vi "Dashboard Main.vi"() -> ()   [LabVIEW 2018]
uses:
  <vilib>/Rock Robotics/WPI/Camera/WPI_CameraExposure Values.ctl
  <vilib>/Rock Robotics/WPI/Camera/WPI_CameraWhite Balance Values.ctl
  <vilib>/Utility/miscctls.llb/LVRowAndColumnTypeDef.ctl
  <vilib>/event_ctls.llb/eventvkey.ctl
  <vilib>/Rock Robotics/Network Tables/NT Read Numeric Array.vi
  <vilib>/Rock Robotics/WPI/Dashboard/WPI_DashboardLogging Global.vi
  Dashboard globals.vi
  <vilib>/vision/NI_Vision_Development_Module.lvlib
panel:
  in  "Camera Settings Right":T1={"Frame Rate"=30, "Compression"=30, "Size"=1, "DB Camera Config"=FALSE} {"Frame Rate" scale=1.0..30.0; "Compression" scale=100.0..-1.0; "Size" items=["640x480", "320x240", "160x120"]}
  in  "Camera Name Right":string(combo)="No Camera Selection"
  out "Camera Perf":string
  in  "Camera Settings":T1={"Frame Rate"=30, "Compression"=30, "Size"=1, "DB Camera Config"=FALSE} {"Frame Rate" scale=1.0..30.0; "Compression" scale=100.0..-1.0; "Size" items=["640x480", "320x240", "160x120"]}
  in  "TCP":refnum<k5>
  in  "Rec Mode":enum32{"Stop", "Record", "Playback"}(radio)
  out "Robot IP":string
  out "Image Message":string="Timeout in Camera Communications"
  in  "Dashboard Tab":T2(tab)=enum."Custom"
  in  "Reset":bool
  out "Total Stored\nSince Reset":i32
  in  "# New Images\nto Store":i32=1
  in  "Photo\nStore Rate":u32=100
  in  "Start\nStoring":bool
  in  "Select Auto":string(combo)="Select Autonomous ..."
  out "NT Connection":bool
  out "MotorChart R":cluster{"Numeric":dbl, "Numeric":dbl}(graph)
  out "MotorChart L":cluster{"Numeric":dbl, "Numeric":dbl}(graph)
  out "MotorSliders R":cluster{"MotorSlide1":dbl, "MotorSlide2":dbl} {"MotorSlide2" scale=-1.0..1.0 scale format="%#_2e"; "MotorSlide1" scale=-1.0..1.0 scale format="%#_2e"}
  out "MotorSliders L":cluster{"MotorSlide1":dbl, "MotorSlide2":dbl} {"MotorSlide2" scale=-1.0..1.0 scale format="%#_2e"; "MotorSlide1" scale=-1.0..1.0 scale format="%#_2e"}
  out "Gyro":dbl(knob) scale=0.0..360.0
  out "JS1 Z":dbl(slide) scale=-1.0..1.0 scale format="%#_2e"
  out "JS1 Graph":cluster{"X":dbl, "Y":dbl}[](graph)
  out "JS1 Buttons":T3
  out "JS2 Z":dbl(slide) scale=-1.0..1.0 scale format="%#_2e"
  out "JS2 Graph":cluster{"X":dbl, "Y":dbl}[](graph)
  out "JS2 Buttons":T3
  out "Mode":T4(ring)=enum."Auto Disabled"
  out "Right Camera Perf":cluster{"Bandwidth (Mbps)":dbl, "FPS":dbl}
  out "Camera Image Right":T5(plugin-control)
  in  "DB/String 9":string
  in  "DB/String 8":string
  in  "DB/String 7":string
  in  "DB/String 6":string
  in  "DB/String 5":string
  in  "DB/String 4":string
  in  "DB/String 3":string
  in  "DB/String 2":string
  in  "DB/String 1":string
  in  "DB/String 0":string
  in  "DB/Slider 0":dbl(slide) scale=0.0..5.0
  in  "DB/Slider 1":dbl(slide) scale=0.0..5.0
  in  "DB/Slider 2":dbl(slide) scale=0.0..5.0
  in  "DB/Slider 3":dbl(slide) scale=0.0..5.0
  out "DB/LED 3":bool
  out "DB/LED 2":bool
  out "DB/LED 1":bool
  out "DB/LED 0":bool
  in  "DB/Button 3":bool
  in  "DB/Button 2":bool
  in  "DB/Button 1":bool
  in  "DB/Button 0":bool caption="New Name"
  out "Right width":sgl
  out "Left width":sgl
  out "Right y":sgl
  out "Right x":sgl
  out "Left y":sgl
  out "Left x":sgl
  out "Right height":sgl
  out "Left height":sgl
  in  "Desired Target":T6(radio)=enum."Ship Right"
  in  "Enable Vision\nProcessing":bool
  in  "Test Slider":dbl(slide) scale=0.0..100.0 scale format="%#_3g"
  in  "On/Off":bool caption="Solenoid"
  in  "Test Name":u16(ring) items=["Select the test to run..."]
  in  "Test Tree":string(tree)
  in  "Motor":cluster{"Value":dbl, "Enable":bool} {"Value" scale=-1.0..1.0 scale format="%#_3g"}
  out "Progress":T7 {"Test Progress" scale=0.0..100.0}
  in  "Rev/Fwd":cluster{"Forward":bool, "Reverse":bool}
  in  "Test Ring":u16(ring) items=["Monochrome", "Color"]
  out "Cmd Status":string
  in  "Execute Command":bool
  in  "Command Params":string[][](table)
  in  "Command Selection":i32(listbox)
  in  "CheckList":i32(listbox)
  out "Tree":string(tree)
  out "Camera Image":T5(plugin-control)
  out "Background":bool
  in  "Camera Name":string(combo)="No Camera Selection"
  # "HW"
  # "HW"
  # "Joysticks"
  # "Drive Motors"
  # "Front"
  # "Right"
  # "Left"
  # "Back"
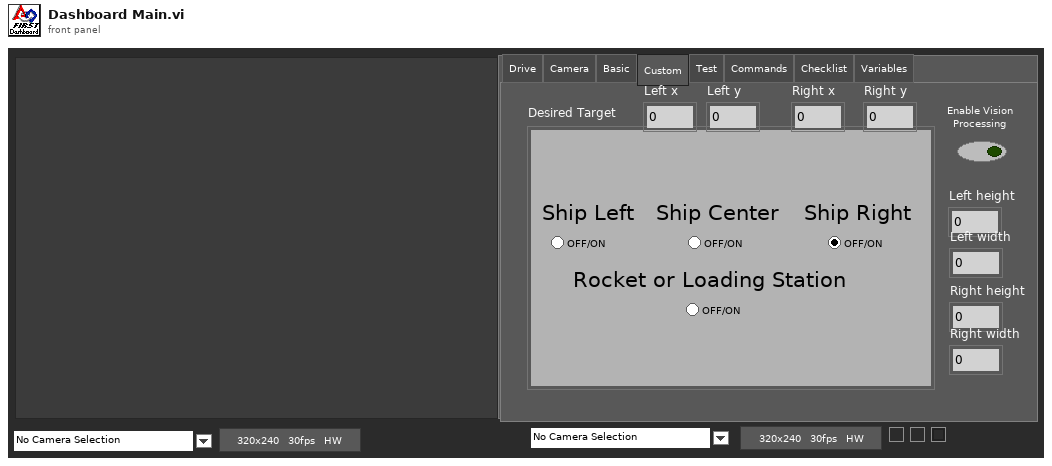
[diagram p1: front panel]
types:
  T1 = cluster{"Frame Rate":i32, "Compression":i32, "Size":u16, "DB Camera Config":bool}
  T2 = enum32{"Drive", "Camera", "Basic", "Custom", "Test", "Commands", "Checklist", "Variables"}
  T3 = cluster{bool, bool, bool, bool, bool, bool, bool, bool, bool, bool, bool, bool}
  T4 = enum8{"Tele-Op Disabled", "Tele-Op Enabled", "Auto Disabled", "Auto Enabled", "Test Disabled", "Test Enabled", "Disconnected", "No Code", "E-Stop"}
  T5 = typedef "IMAQ Image.ctl" = refnum<image>
  T6 = enum32{"Ship Left", "Ship Center", "Ship Right", "Rocket or Loading Station"}
  T7 = cluster{"Test Progress":u8, "Test Progress Text":string}
  T8 = cluster{"Save Path":path, "Interval (s)":dbl, "Keep":i32}
  T9 = typedef "Image Type" = u32
  T10 = cluster{"IDs":cluster{"RPC field ID":u16, "Unique ID":u16}, "String":string}
  T11 = cluster{"Camera Image":refnum<vi>, "Dashboard Tab":refnum<vi>, "Background":refnum<vi>, "Rec Mode":refnum<vi>, "Test Slider":refnum<vi>, "On/Off ":refnum<vi>, "Test Ring":refnum<vi>, "Rev/Fwd":refnum<vi>, "Test Name":refnum<vi>, "Motor":refnum<vi>, "Progress":refnum<vi>, "CheckList":refnum<vi>, "Tree":refnum<vi>, "Test Tree":refnum<vi>, "Command Params":refnum<vi>, "Command Selection":refnum<vi>, "Execute Command":refnum<vi>, "Cmd Status":refnum<vi>, "Camera Settings":refnum<vi>, "Camera Name":refnum<vi>, "Camera Perf":refnum<vi>, "Camera Settings Right":refnum<vi>, "Camera Name Right":refnum<vi>, "Camera Image Right":refnum<vi>}
  T12 = typedef "WPI_CameraExposure Values.ctl" = enum16{"Auto", "Flicker-free 50 Hz", "Flicker-free 60 Hz", "Hold current", "Custom"}
  T13 = typedef "WPI_CameraWhite Balance Values.ctl" = enum16{"Auto", "Fixed indoor", "Fixed outdoor 1", "Fixed outdoor 2", "Fixed fluorescent 1", "Fixed fluorescent 2", "Hold current", "Custom"}
  T14 = cluster{"Exposure":T12, "Exposure (%)":dbl, "Brightness":i32, "White Balance":T13, "Color Temp (K)":dbl}
  T15 = cluster{"Global Rectangle":i32[], "Contours":cluster{"Contour Type":u32, "ROI Type":u32, "Points":i32[]}[]}
  T16 = cluster{"Corners":cluster{"X":sgl, "Y":sgl}[], "Orientation (degrees)":dbl, "Width":dbl, "Height":dbl, "Score":dbl}[]
  T17 = cluster{"Camera Name":string, string, "Saved DB Images Info":cluster{"Save Path":path, "Interval (s)":dbl, "Keep":i32}}
  T18 = cluster{"Corners":cluster{"X":sgl, "Y":sgl}[], "Orientation (degrees)":dbl, "Width":dbl, "Height":dbl, "Score":dbl}
  T19 = cluster{"Corners[0]":cluster{"X":sgl, "Y":sgl}, "Corners[1]":cluster{"X":sgl, "Y":sgl}, "Corners[2]":cluster{"X":sgl, "Y":sgl}, "Corners[3]":cluster{"X":sgl, "Y":sgl}, "Corners[4]":cluster{"X":sgl, "Y":sgl}, "Corners[5]":cluster{"X":sgl, "Y":sgl}, "Corners[6]":cluster{"X":sgl, "Y":sgl}, "Corners[7]":cluster{"X":sgl, "Y":sgl}, "Corners[8]":cluster{"X":sgl, "Y":sgl}}
  T20 = cluster{"Camera Name Right":string, string, "Saved DB Images Info":cluster{"Save Path":path, "Interval (s)":dbl, "Keep":i32}}
  T21 = cluster{"Error Strings":string, "Disable Counts":cluster{u16, u16}, "Rail Faults":cluster{u16, u16, u16}, "Robot IP":string, "DB Mode":u8, "Event Info":cluster{"Name":string, "Type":u8, "Number":u16, "Replay":u8}}
  T22 = cluster{"Storage":cluster{"Disk Free":u64, "RAM Block":u32, "RAM free":u32}, "CPU Utilization":cluster{"CPU % ISR":sgl, "CPU % Time Crit":sgl, "CPU % Timed Str":sgl, "CPU % High":sgl, "CPU % Above":sgl, "CPU % Normal":sgl, "CPU % Low":sgl}, "CAN":cluster{"% Bus Utilization":sgl, "Bus Off Cnt":u32, "TX_FIFO Full Cnt":u32, "Receive Error Cnt":u8, "Transmit Error Cnt":u8}, "HID":cluster{"HID Outputs":u32, "Rumble Low":u16, "Rumble High":u16}[]}
  T23 = cluster{"Status bits":cluster{"Test Mode":bool, "Autonomous":bool, "Enabled":bool, "Code Start":bool, "Brownout":bool, "Reserved 2":bool, "Reserved 3":bool, "E-Stop":bool}, "Code Trace":cluster{"Disabled":bool, "TeleOp":bool, "Auto":bool, "Test":bool}, "Controller Type":enum16{"unknown", "cRIO", "roboRio"}, "Code?":enum16{"unknown", "noCode", "code"}, "Battery V":dbl}
  T24 = cluster{"Control Bits":cluster{"TestMode":bool, "Autonomous":bool, "Enabled":bool, "FMS Present":bool, bool, bool, bool, "E-Stop":bool}, "Team Station ":u8, "Countdown":sgl, "Joystick Values":cluster{"Axes":dbl[], "Buttons":bool[], "POVs":i16[]}[]}
  T25 = cluster{"Axes":dbl[], "Buttons":bool[], "POVs":i16[]}[]
  T26 = cluster{"Axes":dbl[], "Buttons":bool[], "POVs":i16[]}
  T27 = cluster{"Buttons[0]":bool, "Buttons[1]":bool, "Buttons[2]":bool, "Buttons[3]":bool, "Buttons[4]":bool, "Buttons[5]":bool, "Buttons[6]":bool, "Buttons[7]":bool, "Buttons[8]":bool, "Buttons[9]":bool, "Buttons[10]":bool, "Buttons[11]":bool}
  T28 = cluster{"Operation":enum16{"Update", "Clear"}, "Color Box":u32}[]
  T29 = typedef "eventvkey.ctl" = enum16{"ASCII", "Enter", "Return", "Shift", "Ctrl", "Alt", "Cmd", "Opt", "Caps", "NumLock", "Clear", "Break", "Up", "Down", "Left", "Right", "Insert", "Delete", "Home", "End", "PageUp", "PageDown", "Escape", "Help", "Pause", "ScrollLock", "F1", "F2", "F3", "F4", "F5", "F6", "F7", "F8", "F9", "F10", "F11", "F12", "F13", "F14", "F15", "F16", "F17", "F18", "F19", "F20", "F21", "F22", "F23", "F24", "Play", "VolumeUp", "VolumeDown", "Mute", "Two Byte Char"}
  T30 = cluster{"Image Size":bool, "Image Type":bool, "Pixel Value":bool, "ROI Information":bool, "Zoom Factor":bool}
  T31 = cluster{"Operation":enum16{"Update", "Clear"}, "Color Box":u32}
  T32 = typedef "LVRowAndColumnTypeDef.ctl" = cluster{"Row":i32, "Column":i32}
  T33 = cluster{"Shift":bool, "Ctrl":bool, "Alt":bool, "Cmd":bool, "Opt":bool}
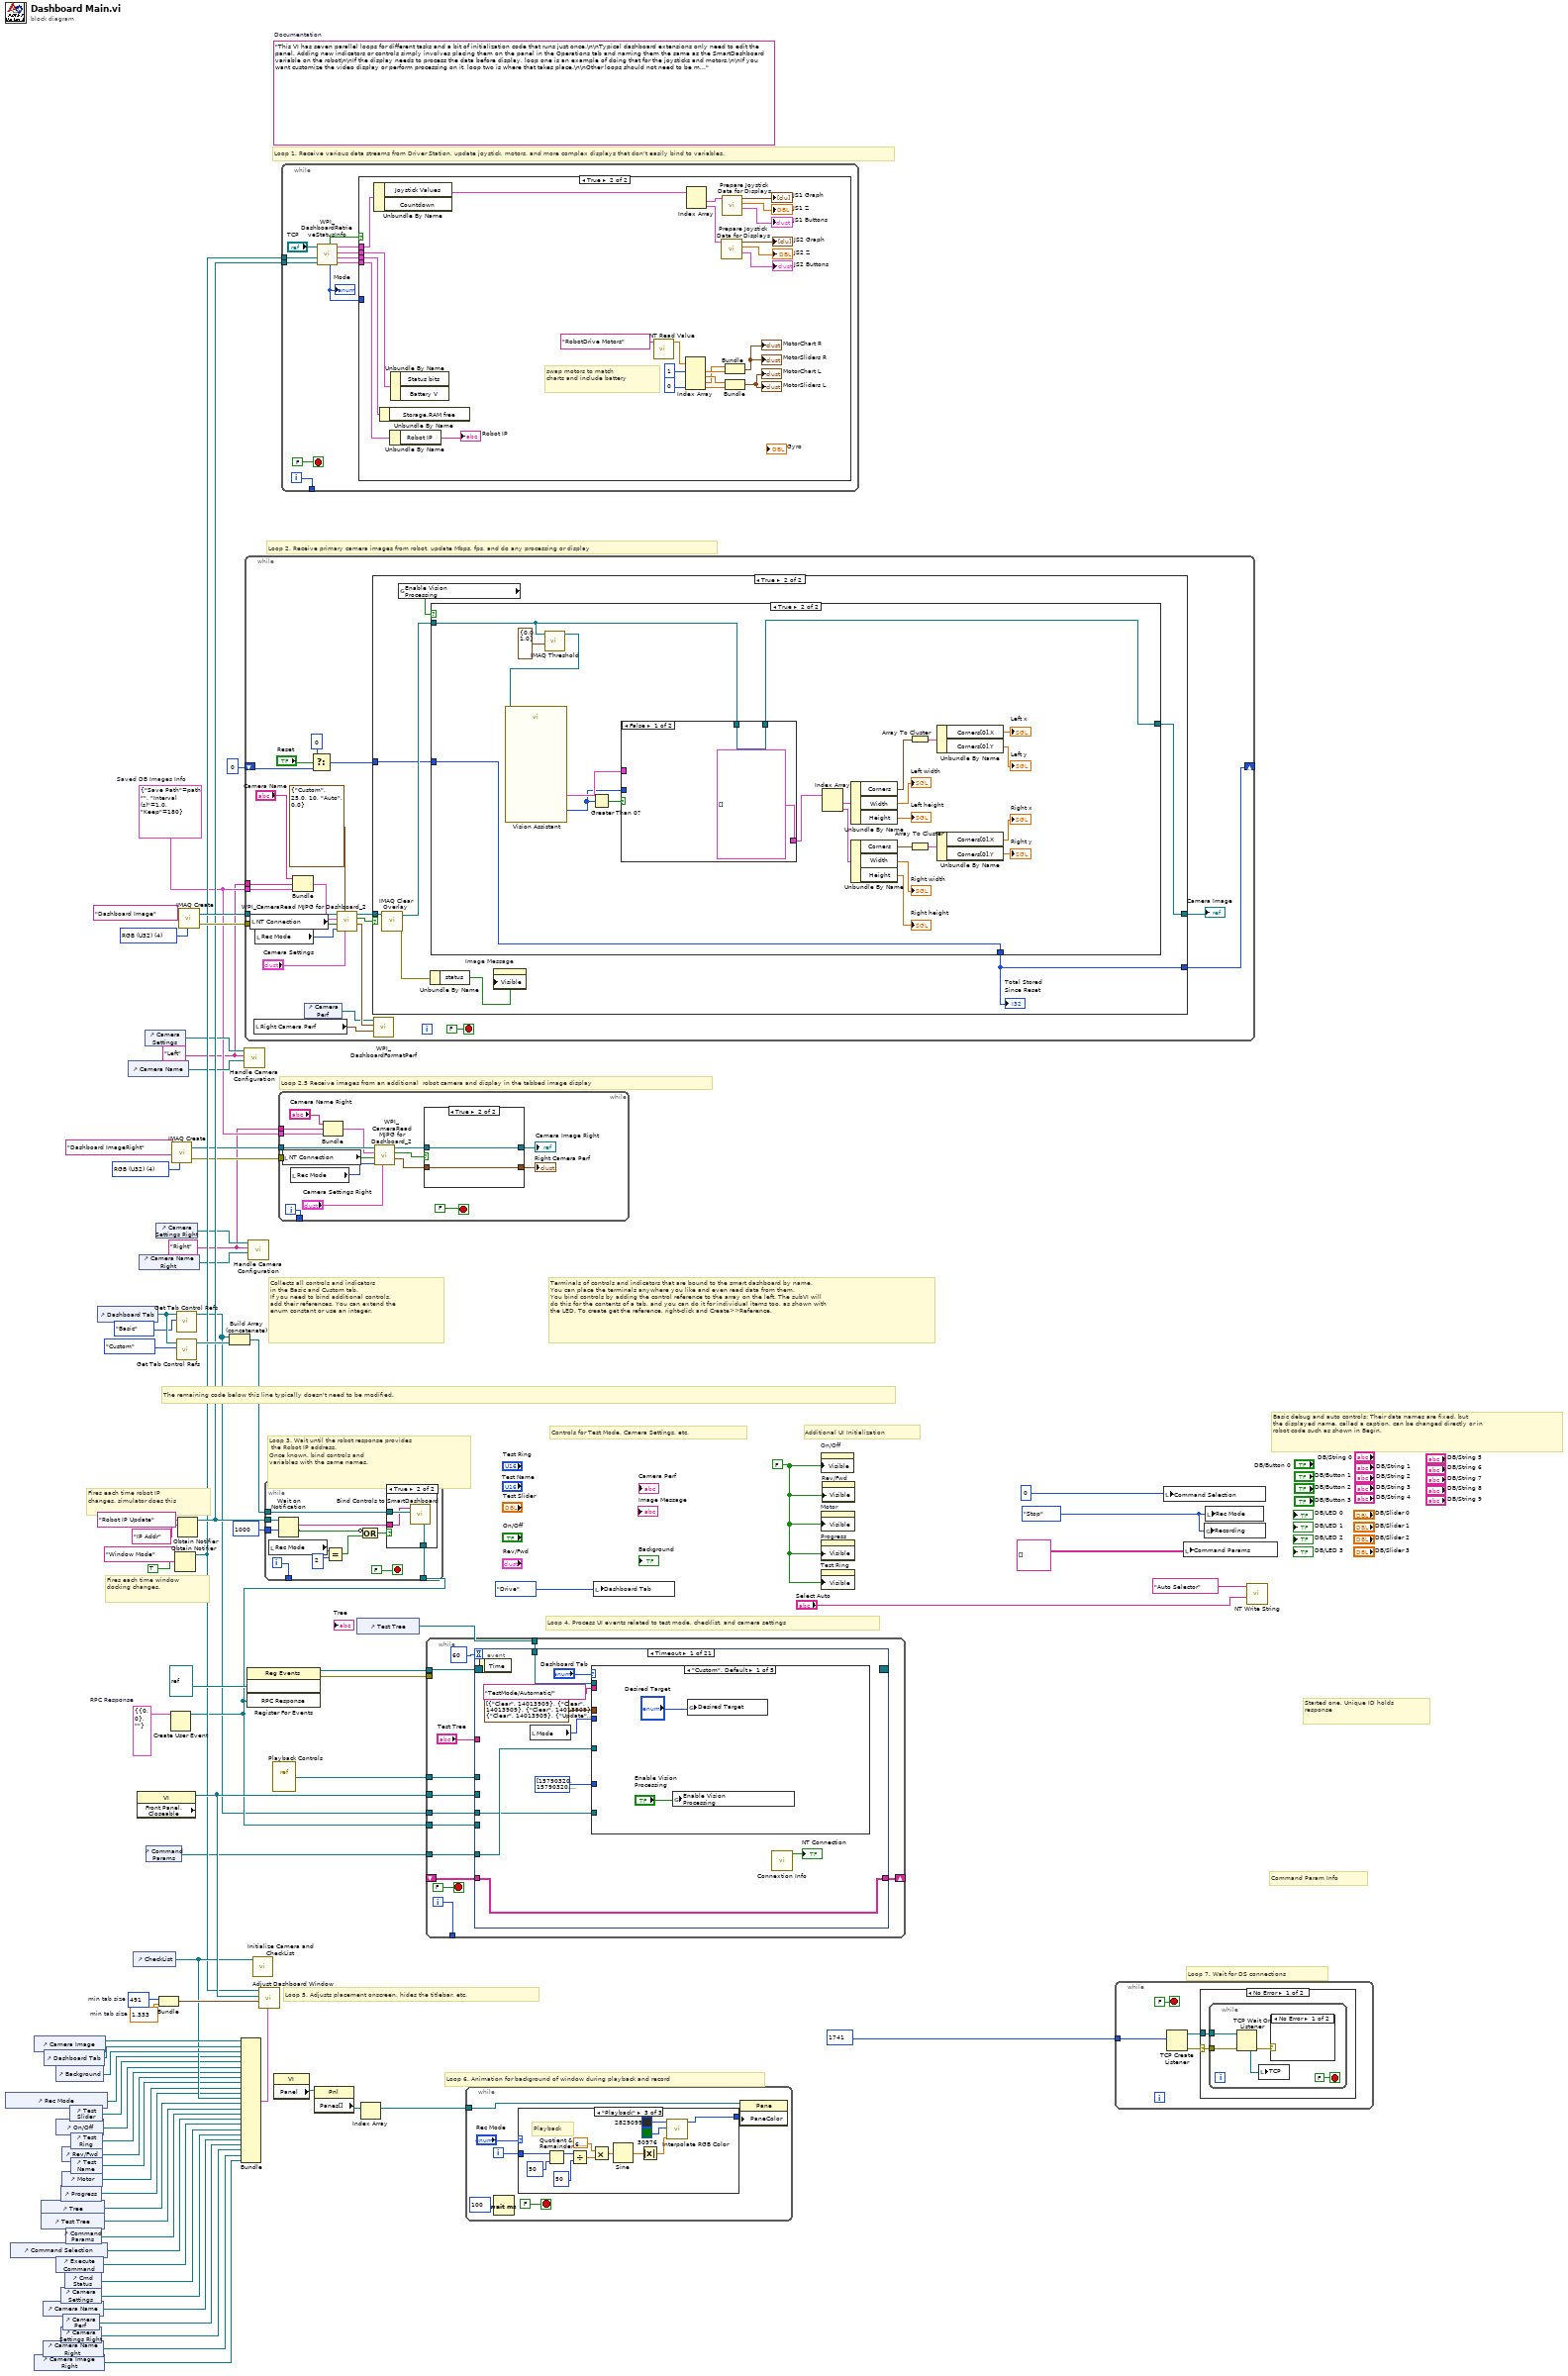
[diagram p0: block diagram]
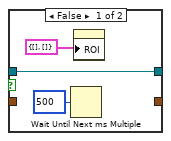
[diagram p2: hidden frame]
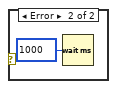
[diagram p3: hidden frame]
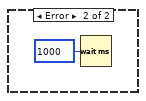
[diagram p4: hidden frame]
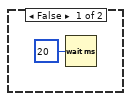
[diagram p5: hidden frame]
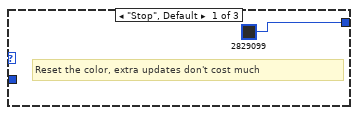
[diagram p6: hidden frame]
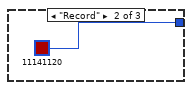
[diagram p7: hidden frame]
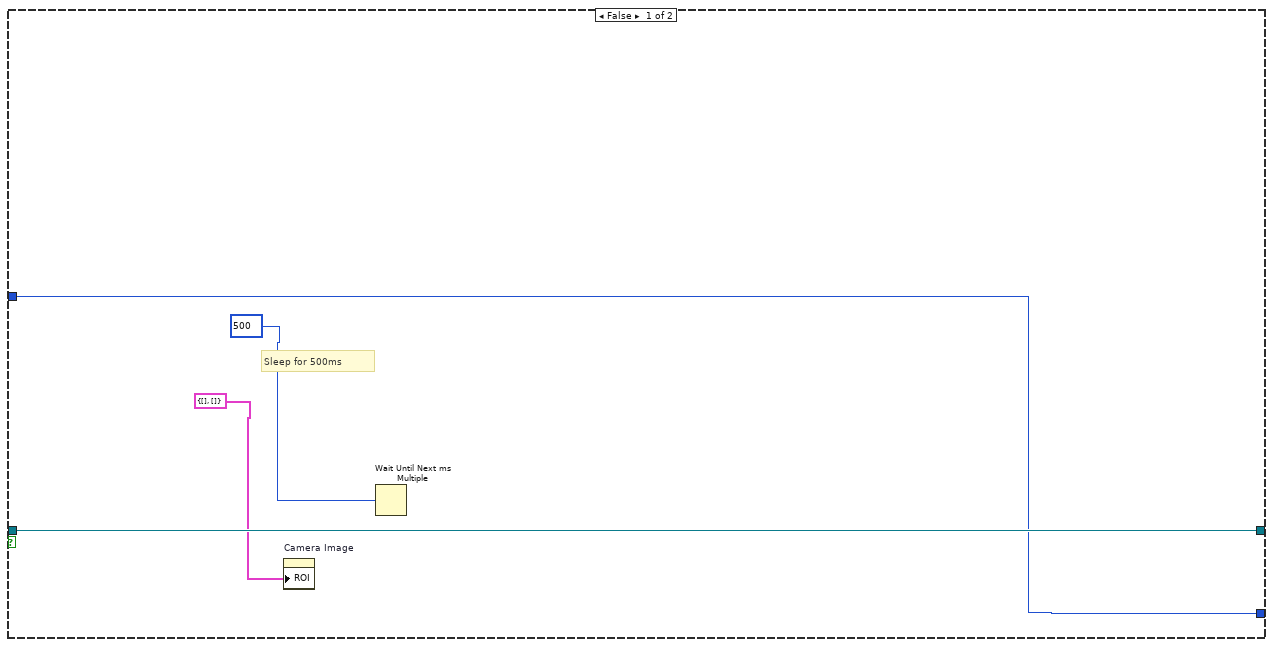
[diagram p9: hidden frame]
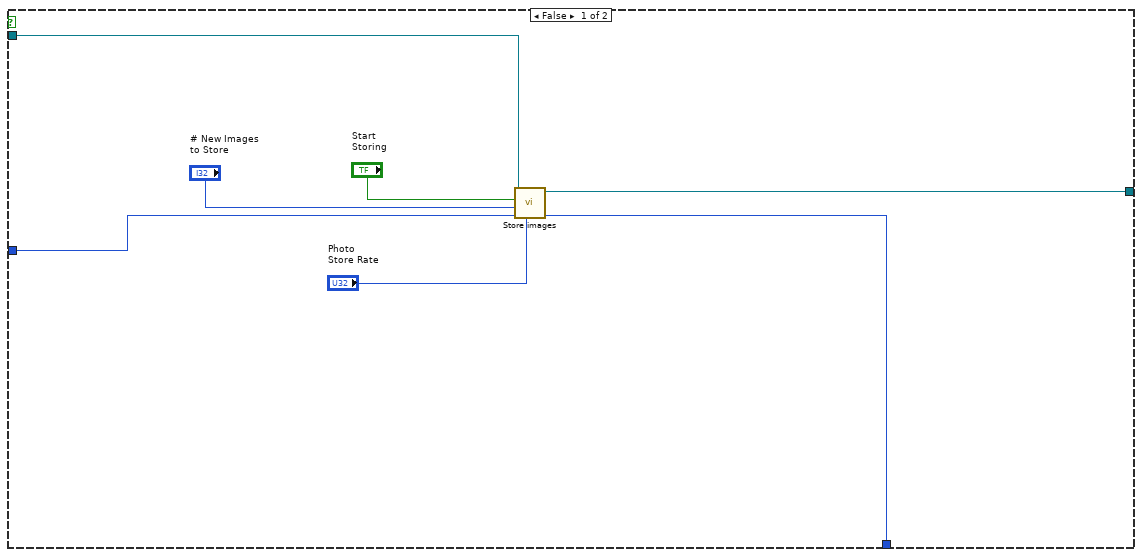
[diagram p10: hidden frame]
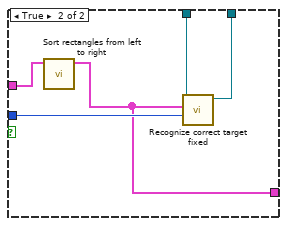
[diagram p11: hidden frame]
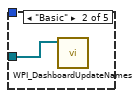
[diagram p12: hidden frame]
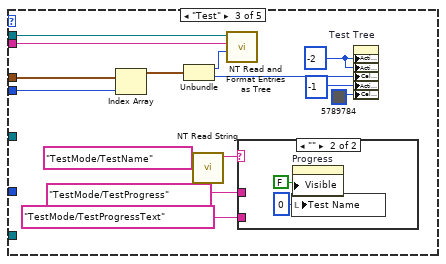
[diagram p13: hidden frame]
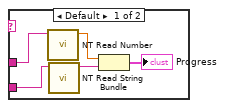
[diagram p14: hidden frame]
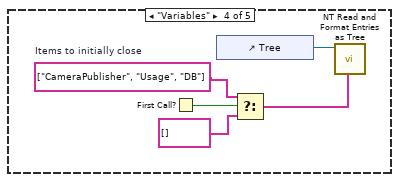
[diagram p15: hidden frame]
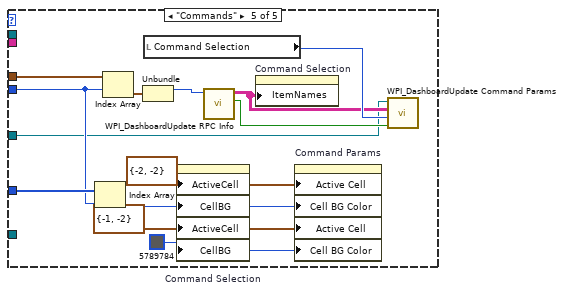
[diagram p16: hidden frame]
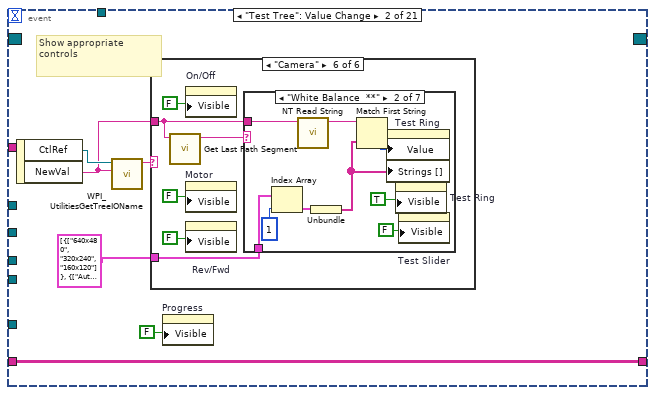
[diagram p17: hidden frame]
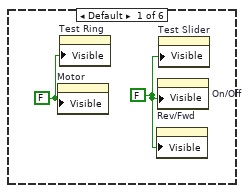
[diagram p18: hidden frame]
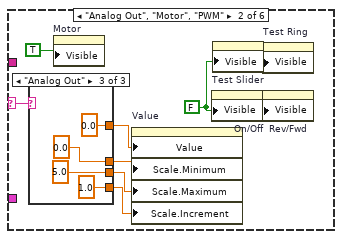
[diagram p19: hidden frame]
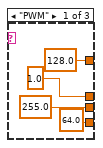
[diagram p20: hidden frame]
diagram:
  w4 = T8 {"Save Path"=path "", "Interval (s)"=1.0, "Keep"=180}  # Saved DB Images Info
  w3 = "Right"
  w2 = "Left"
  w14 = T9 4 items=["Grayscale (U8)", "Grayscale (I16)", "Grayscale (SGL)", "Complex (CSG)", "RGB (U32)", "HSL (U32)", "RGB (U64)"] ("Image Type")
  w30 = T10 {"IDs"={"RPC field ID"=0, "Unique ID"=0}, "String"=""}  # RPC Response
  w53 = 491  # min tab size
  w52 = 1.333  # min tab size
  w60 = enum32{"Stop", "Record", "Playback"}."Stop" ("Rec Mode")
  w37 = FALSE ("Visible")
  (unwired) "This VI has seven parallel loops for different tasks and a bit of initialization code that runs just once.\n\nTypical dashboard extensions only need to edit the panel. Adding new indicators or controls simply involves placing them on the panel in the Operations tab and naming them the same as the SmartDashboard variable on the robot\n\nIf the display needs to process the data before display, loop one is an example of doing that for the joysticks and motors.\n\nIf you want customize the video display or perform processing on it, loop two is where that takes place.\n\nOther loops should not need to be modified. They are pretty standard, and document the task they perform."  # Documentation
  w77 = T9 4 items=["Grayscale (U8)", "Grayscale (I16)", "Grayscale (SGL)", "Complex (CSG)", "RGB (U32)", "HSL (U32)", "RGB (U64)"] ("Image Type")
  # "Loop 2.5 Receive images from an additional  robot camera and display in the tabbed image display"
  # "Command Param Info"
  # "Started one, Unique ID holds\nresponse"
  # "Loop 7. Wait for DS connections"
  # "Basic debug and auto controls: Their data names are fixed, but\nthe displayed name, called a caption, can be changed directly or in\nrobot code such as shown in Begin."
  # "Controls for Test Mode, Camera Settings, etc."
  # "Additional UI Initialization"
  # "Loop 6. Animation for background of window during playback and record"
  # "Fires each time robot IP\nchanges, simulator does this"
  # "Fires each time window\ndocking changes."
  # "Collects all controls and indicators\nin the Basic and Custom tab.\nIf you need to bind additional controls,\nadd their references. You can extend the\nenum constant or use an integer."
  # "The remaining code below this line typically doesn't need to be modified."
  # "Loop 4. Process UI events related to test mode, checklist, and camera settings"
  # "Terminals of controls and indicators that are bound to the smart dashboard by name.\nYou can place the terminals anywhere you like and even read data from them.\nYou bind controls by adding the control reference to the array on the left. The subVI will\ndo this for the contents of a tab, and you can do it for individual items too, as shown with\nthe LED. To create get the reference, right-click and Create>>Reference."
  # "Loop 3. Wait until the robot response provides\n the Robot IP address.\nOnce known, bind controls and\nvariables with the same names."
  # "Loop 5. Adjusts placement onscreen, hides the titlebar, etc."
  # "Loop 1. Receive various data streams from Driver Station, update joystick, motors, and more complex displays that don't easily bind to variables."
  # "Loop 2. Receive primary camera images from robot, update Mbps, fps, and do any processing or display"
  n1 = control-ref of="Rec Mode"() -> (w43:refnum<vi>)
  n2 = control-ref of="Command Selection"() -> (w29:refnum<vi>)
  n3 = control-ref of="Camera Image Right"() -> (w7:refnum<vi>)
  n4 = control-ref of="Camera Image"() -> (w55:refnum<vi>)
  n5 = control-ref of="Tree"() -> (w47:refnum<vi>)
  n6 = control-ref of="Test Tree"() -> (w46:refnum<vi>)
  n7 = control-ref of="Camera Name"() -> (w20:refnum<vi>)
  n8 = control-ref of="Camera Name Right"() -> (w8:refnum<vi>)
  n9 = control-ref of="Dashboard Tab"() -> (w54:refnum<vi>)
  n10 = control-ref of="Execute Command"() -> (w31:refnum<vi>)
  n11 = control-ref of="Background"() -> (w50:refnum<vi>)
  n12 = control-ref of="On/Off"() -> (w41:refnum<vi>)
  n13 = control-ref of="Progress"() -> (w38:refnum<vi>)
  n14 = control-ref of="Camera Settings"() -> (w21:refnum<vi>)
  n15 = control-ref of="Camera Settings Right"() -> (w9:refnum<vi>)
  n16 = control-ref of="Rev/Fwd"() -> (w39:refnum<vi>)
  n17 = control-ref of="Motor"() -> (w44:refnum<vi>)
  n18 = control-ref of="Camera Perf"() -> (w19:refnum<vi>)
  n19 = control-ref of="Cmd Status"() -> (w25:refnum<vi>)
  n20 = control-ref of="Command Params"() -> (w32:refnum<vi>)
  n21 = control-ref of="Test Slider"() -> (w42:refnum<vi>)
  n22 = control-ref of="Test Ring"() -> (w40:refnum<vi>)
  n23 = control-ref of="Test Name"() -> (w45:refnum<vi>)
  n24 = control-ref of="Dashboard Tab"() -> (w58:refnum<vi>)
  n25 = control-ref of="Camera Name"() -> (w22:refnum<vi>)
  n26 = control-ref of="CheckList"() -> (w48:refnum<vi>)
  n27 = property class="VI" props=["Front Panel.Closeable"]() -> (reference out=w59:refnum<vi>)  [unwired: 2 in, 2 out]
  n28 = control-ref of="Camera Name Right"() -> (w10:refnum<vi>)
  n29 = control-ref of="Camera Settings"() -> (w23:refnum<vi>)
  n30 = control-ref of="Command Params"() -> (w24:refnum<vi>)
  n31 = control-ref of="Camera Settings Right"() -> (w11:refnum<vi>)
  n32 = Bundle("min tab size"=w53, "min tab size"=w52) -> (w51:cluster{"min tab size":i32, "min tab size":dbl})  [unwired: 1 in]
  n33 = Create User Event(user event datatype=w30) -> (user event=w26:refnum<user-event>)  [unwired: 1 in, 1 out]
  n34 = call "IMAQ Create"("Image Name"="Dashboard ImageRight", "Image Type"=w14) -> ("New Image"=w13:T5, "error out"=w12:errorcluster)  [unwired: 2 in, 1 out]
  n35 = Obtain Notifier(name (unnamed)="Window Mode", notification data type=TRUE) -> (notifier out=w35:refnum<notifier>)  [unwired: 2 in, 2 out]
  n36 = call <vilib>:"Get Tab Control Refs.vi"("Page Index"=T2."Basic" ("Dashboard Tab"), "TabControl in"=w58) -> ("ControlsOnPage"=w18:refnum<vi>[])  [unwired: 9 in]
  n37 = call <vilib>:"Get Tab Control Refs.vi"("Page Index"=T2."Custom" ("Dashboard Tab"), "TabControl in"=w58) -> ("ControlsOnPage"=w57:refnum<vi>[])  [unwired: 9 in]
  n38 = Obtain Notifier(name (unnamed)="Robot IP Update", notification data type="IP Addr" ("name (unnamed)")) -> (notifier out=w36:refnum<notifier>)  [unwired: 2 in, 2 out]
  n39 = call "IMAQ Create"("Image Name"="Dashboard Image", "Image Type"=w77) -> ("New Image"=w75:T5, "error out"=w74:errorcluster)  [unwired: 2 in, 1 out]
  n40 = Build Array (concatenate)(w18, w57) -> (w56:refnum<vi>[])
  n41 = Bundle("Camera Image"=w55, "Dashboard Tab"=w54, "Background"=w50, "Rec Mode"=w43, "Test Slider"=w42, "On/Off"=w41, "Test Ring"=w40, "Rev/Fwd"=w39, "Test Name"=w45, "Motor"=w44, "Progress"=w38, "CheckList"=w48, "Tree"=w47, "Test Tree"=w46, "Command Params"=w32, "Command Selection"=w29, "Execute Command"=w31, "Cmd Status"=w25, "Camera Settings"=w21, "Camera Name"=w20, "Camera Perf"=w19, "Camera Settings Right"=w9, "Camera Name Right"=w8, "Camera Image Right"=w7) -> (w49:T11)  [unwired: 1 in]
  n42 = call "Handle Camera Configuration.vi"("CameraNameRef"=w22, "Display Name"=w2, "ClusterRef"=w23) -> ()  [unwired: 9 in]
  n43 = while {
    tunnel: w75 -> [w97]
    tunnel: w74 -> [_]
    tunnel: w4 -> [w90]
    tunnel: w2 -> [w87]
    shift-right: [w79] -> _
    shift-left: 0 -> [w82]
    stop <- FALSE stop-if-true
    n44 = local read "NT Connection"() -> (w91:bool)
    n45 = local read "Right Camera Perf"() -> (w85:cluster{"Bandwidth (Mbps)":dbl, "FPS":dbl})
    n46 = local read "Rec Mode"() -> (w94:enum32{"Stop", "Record", "Playback"})
    n47 = Bundle("Camera Name"="Camera Name", w87, "Saved DB Images Info"=w90) -> (w89:T17)  [unwired: 1 in]
    n48 = control-ref of="Camera Perf"() -> (w84:refnum<vi>)
    n49 = Select(t=0, s="Reset", f=w82) -> (s? t:f=w80:i32)
    n50 = call <vilib>:"WPI_CameraRead MJPG for Dashboard_2.vi"("Camera Settings"="Camera Settings", "Camera Settings 2"=T14 {"Exposure"=enum."Custom", "Exposure (%)"=25.0, "Brightness"=10, "White Balance"=enum."Auto", "Color Temp (K)"=0.0}, "Rec Mode"=w94, "NT Connection"=w91, "Capture Info"=w89, "Image in"=w97) -> ("perf info"=w86:cluster{"Bandwidth (Mbps)":dbl, "fps":dbl}, "Active"=w95:bool, "Image\\ out"=w96:T5)  [unwired: 3 in]
    n51 = case shown="True" w95 {
      tunnel: w96 -> [w101 w108]
      tunnel: [w101 w105] -> w92
      tunnel: w80 -> [w99 w106]
      tunnel: [w99 w104] -> w79
      frame False {
        # "Sleep for 500ms"
        n52 = property on="Camera Image" class="ImageControl"("ROI"=T15 {"Global Rectangle"=[], "Contours"=[]}) -> ()  [unwired: 2 in, 2 out]
        n53 = Wait Until Next ms Multiple(millisecond multiple=u32 500) -> ()  [unwired: 1 out]
      }
      frame True {
        n54 = call "IMAQ Clear Overlay"("Image"=w108) -> ("error out"=w109:errorcluster, "Image Out"=w107:T5)  [unwired: 2 in, 7 out]
        n55 = global read "Dashboard globals.vi" "Enable Vision\nProcessing"() -> (w103:bool)
        n56 = Unbundle By Name(w109) -> ("status"=w110:bool)
        n57 = case shown="True" w103 {
          tunnel: w107 -> [w114 w137]
          tunnel: w106 -> [w113 w140]
          tunnel: [w112 w139] -> w105
          tunnel: [w111 w140] -> w104
          frame False {
            n58 = call "Store images.vi"("ms Capture Rate"="Photo\nStore Rate", "# Total images IN"=w113, "# new images to capture"="# New Images\nto Store", "Store # Images?"="Start\nStoring", "Image"=w114) -> ("Total images OUT"=w111:i32, "Image Out"=w112:T5)  [unwired: 5 in]
          }
          frame True {
            n59 = call "IMAQ Threshold"("Range"=cluster{"Lower value":sgl, "Upper value":sgl} {"Lower value"=0.0, "Upper value"=1.0}, "Image Src"=w137) -> ("Image Dst Out"=w136:T5)  [unwired: 8 in, 1 out]
            n60 = call "Vision Assistant"("Image In"=w136) -> ("Number of Matches (Shape Detection 1)"=w133:i32, "Rectangles Calibrated (Shape Detection 1)"=w134:T16)  [unwired: 23 in, 2 out]
            n61 = Greater Than 0?(x=w133) -> (x > 0?=w135:bool)
            n62 = case shown="False" w135 {
              tunnel: [w142 w147] -> w139
              tunnel: w137 -> [w142 w146]
              tunnel: w134 -> [_ w145]
              tunnel: w133 -> [_ w144]
              tunnel: [T16 [] ("Rectangles (Calibrated) OUT") w143] -> w132
              frame False {
              }
              frame True {
                n63 = call "Sort rectangles from left to right.vi"("Rectangles (Calibrated) IN"=w145) -> ("Rectangles (Calibrated) OUT"=w143:T16)  [unwired: 10 in]
                n64 = call "Recognize correct target fixed.vi"("# rectangles"=w144, "Rectangles (Calibrated)"=w143, "Image"=w146) -> ("Image Out"=w147:T5)  [unwired: 8 in]
              }
            }
            n65 = Index Array(array=w132) -> (element #1=w126:T18, element #2=w131:T18)  [unwired: 2 in]
            n66 = Unbundle By Name(w126) -> ("Corners"=w127:cluster{"X":sgl, "Y":sgl}[], "Width"=→"Left width":dbl, "Height"=→"Left height":dbl)
            n67 = Unbundle By Name(w131) -> ("Corners"=w130:cluster{"X":sgl, "Y":sgl}[], "Width"=→"Right width":dbl, "Height"=→"Right height":dbl)
            n68 = Array To Cluster(array=w127) -> (cluster=w128:T19)
            n69 = Array To Cluster(array=w130) -> (cluster=w129:T19)
            n70 = Unbundle By Name(w128) -> ("Corners[0].X"=→"Left x":sgl, "Corners[0].Y"=→"Left y":sgl)
            n71 = Unbundle By Name(w129) -> ("Corners[0].X"=→"Right x":sgl, "Corners[0].Y"=→"Right y":sgl)
          }
        }
        "Total Stored\nSince Reset" <- w104
        n72 = property on="Image Message" class="Str"("Visible"=w110) -> ()  [unwired: 2 in, 2 out]
      }
    }
    "Camera Image" <- w92
    n73 = call <vilib>:"WPI_DashboardFormatPerf.vi"("Right Camera Perf"=w85, "Performance"=w86, "String in"=w84) -> ()  [unwired: 9 in]
  }
  n74 = register-events(refnum<vi> refnum, w26) -> (reference out=w64:refnum<event-registration>, error out=w63:errorcluster)  [unwired: 2 in]
  n75 = call "Handle Camera Configuration.vi"("CameraNameRef"=w10, "Display Name"=w3, "ClusterRef"=w11) -> ()  [unwired: 9 in]
  n76 = call "Initialize Camera and CheckList.vi"("ListBox in"=w48) -> ()  [unwired: 11 in]
  n77 = call "Adjust Dashboard Window.vi"("Sizing Refnums"=w49, "Size Constraints"=w51, "VI"=w59, "WIn Mode"=w35) -> ()  [unwired: 8 in]
  n78 = while {
    tunnel: w56 -> [w159]
    tunnel: w36 -> [w157]
    tunnel: [w155] -> _
    tunnel: u32 1000 ("milliseconds to wait") -> [w154]
    tunnel: w26 -> [w148]
    i -> [w155]
    stop <- FALSE stop-if-true
    n79 = local read "Rec Mode"() -> (w150:enum32{"Stop", "Record", "Playback"})
    n80 = Wait on Notification(notifier=w157, timeout in ms (-1)=w154) -> (notification=w156:string, timed out?=w152:bool)  [unwired: 2 in, 2 out]
    n81 = Equal?(x=w150, y=u16 2 ("Rec Mode")) -> (x = y?=w151:bool)
    n82 = Compound Arithmetic op=OR(invert w152, w151) -> (w153:bool)
    n83 = case shown="True" w153 {
      tunnel: w159 -> [_ w162]
      tunnel: w156 -> [_ w161]
      tunnel: w148 -> [_ w160]
      frame False {
      }
      frame True {
        n84 = call <vilib>:"Bind Controls to SmartDashboard.vi"("RPC ref"=w160, "Bound Control Refs"=w162, "Server IP Address"=w161) -> ()  [unwired: 9 in]
      }
    }
  }
  n85 = vi-ref "Playback Controls.vi"() -> (w65:refnum<vi>)
  n86 = property class="VI"() -> ("Panel"=w67:refnum<vi>)  [unwired: 2 in, 2 out]
  n87 = while {
    tunnel: w13 -> [w177]
    tunnel: w12 -> [_]
    tunnel: [w172] -> _
    tunnel: w4 -> [w168]
    tunnel: w3 -> [w165]
    i -> [w172]
    stop <- FALSE stop-if-true
    n88 = local read "NT Connection"() -> (w169:bool)
    n89 = local read "Rec Mode"() -> (w176:enum32{"Stop", "Record", "Playback"})
    n90 = Bundle("Camera Name Right"="Camera Name Right", w165, "Saved DB Images Info"=w168) -> (w167:T20)  [unwired: 1 in]
    n91 = call <vilib>:"WPI_CameraRead MJPG for Dashboard_2.vi"("Camera Settings"="Camera Settings Right", "Rec Mode"=w176, "NT Connection"=w169, "Capture Info"=w167, "Image in"=w177) -> ("perf info"=w163:cluster{"Bandwidth (Mbps)":dbl, "fps":dbl}, "Active"=w171:bool, "Image\\ out"=w174:T5)  [unwired: 4 in]
    n92 = case shown="True" w171 {
      tunnel: w174 -> [w179 w182]
      tunnel: [w179 w182] -> w170
      tunnel: [_ w181] -> w164
      tunnel: w163 -> [_ w181]
      frame False {
        n93 = Wait Until Next ms Multiple(millisecond multiple=u32 500) -> ()  [unwired: 1 out]
        n94 = property on="Camera Image Right" class="ImageControl"("ROI"=T15 {"Global Rectangle"=[], "Contours"=[]}) -> ()  [unwired: 2 in, 2 out]
      }
      frame True {
      }
    }
    "Camera Image Right" <- w170
    "Right Camera Perf" <- w164
  }
  n95 = while {
    tunnel: [w192] -> _
    tunnel: w36 -> [w186]
    tunnel: w35 -> [w183]
    i -> [w192]
    stop <- FALSE stop-if-true
    n96 = call <vilib>:"WPI_DashboardRetrieveStatusInfo.vi"("Binding Refnum"=w186, "Window Mode Notifier"=w183, "TCP Cnx"="TCP") -> ("Power and Errors"=w187:T21, "Robot Metrics"=w190:T22, "Status Info"=w191:T23, "Control Info"=w188:T24, "Robot Mode"=w185:T4, "Process?"=w189:bool)  [unwired: 3 in]
    "Mode" <- w185
    n97 = case shown="True" w189 {
      tunnel: w191 -> [_ w218]
      tunnel: w190 -> [_ w217]
      tunnel: w188 -> [_ w216]
      tunnel: w187 -> [_ w215]
      tunnel: w185 -> [_ _]
      frame False {
        n98 = Wait (ms)(milliseconds to wait=u32 20) -> ()  [unwired: 1 out]
      }
      frame True {
        # "swap motors to match\ncharts and include battery"
        n99 = Unbundle By Name(w216) -> ("Joystick Values"=w206:T25)  [unwired: 1 out]
        n100 = Unbundle By Name(w217) -> ()  [unwired: 1 out]
        n101 = Unbundle By Name(w215) -> ("Robot IP"=→"Robot IP":string)
        n102 = Unbundle By Name(w218) -> ()  [unwired: 2 out]
        n103 = call-poly <vilib>:"NT Read Value.vi"("Name"="RobotDrive Motors") -> ("Numeric Array"=w196:dbl[])  [unwired: 9 in, 1 out]
        n104 = Index Array(array=w196, index #1=1, index #4=0) -> (element #1=w210:dbl, element #2=w211:dbl, element #3=w209:dbl, element #4=w214:dbl)  [unwired: 2 in]
        n105 = Index Array(array=w206) -> (element #1=w205:T26, element #2=w201:T26)  [unwired: 2 in]
        n106 = call "Prepare Joystick Data for Displays.vi"("Joystick Values"=w201) -> ("Buttons"=→"JS2 Buttons":T27, "Z Axis"=→"JS2 Z":dbl, "Cartesian Data"=→"JS2 Graph":cluster{"X axis":dbl, "X axis":dbl}[])  [unwired: 8 in]
        n107 = call "Prepare Joystick Data for Displays.vi"("Joystick Values"=w205) -> ("Buttons"=→"JS1 Buttons":T27, "Z Axis"=→"JS1 Z":dbl, "Cartesian Data"=→"JS1 Graph":cluster{"X axis":dbl, "X axis":dbl}[])  [unwired: 8 in]
        n108 = Bundle("Numeric"=w209, "Numeric"=w210) -> (→"MotorChart R" →"MotorSliders R":cluster{"Numeric":dbl, "Numeric":dbl})  [unwired: 1 in]
        n109 = Bundle("Numeric"=w211, "Numeric"=w214) -> (→"MotorChart L" →"MotorSliders L":cluster{"Numeric":dbl, "Numeric":dbl})  [unwired: 1 in]
      }
    }
  }
  n110 = property class="Pnl"(reference=w67) -> ("Panes[]"=w68:refnum<vi>[])  [unwired: 1 in, 2 out]
  n111 = control-ref of="Test Tree"() -> (w69:refnum<vi>)
  n112 = Index Array(array=w68) -> (element=w66:refnum<vi>)  [unwired: 1 in]
  n113 = while {
    tunnel: [w228] -> _
    tunnel: w69 -> [w227]
    tunnel: w65 -> [w226]
    tunnel: w64 -> [w225]
    tunnel: w63 -> [_]
    tunnel: w59 -> [w224]
    tunnel: w26 -> [w223]
    tunnel: w24 -> [w222]
    shift-right: [w221] -> _
    shift-left: _ -> [w220]
    tunnel: w18 -> [w219]
    i -> [w228]
    stop <- FALSE stop-if-true
    n114 = event shown="[0] Timeout" {
      selector: w225 -> [_ _ _ _ _ _ _ _ _ _ _ _ _ _ _ _ _ _ _ _ _]
      dyn-events: [_ _ _ _ _ _ _ _ _ _ _ _ _ _ _ _ w490 _ _ _ _] -> _
      timeout: u32 60 ("milliseconds to wait") -> [_ _ _ _ _ _ _ _ _ _ _ _ _ _ _ _ _ _ _ _ _]
      tunnel: w227 -> [w240 _ _ _ _ _ _ _ _ _ _ _ _ _ _ _ _ _ _ _ _]
      tunnel: "Test Tree" -> [_ _ _ _ _ _ _ _ _ _ _ w457 w465 w467 w471 w479 _ _ _ _ _]
      tunnel: w226 -> [_ _ _ _ _ _ _ _ _ _ _ _ _ _ _ _ w492 _ w510 _ _]
      tunnel: w224 -> [_ _ _ _ _ _ _ _ _ _ _ _ _ _ _ _ w488 _ _ _ _]
      tunnel: w223 -> [_ _ _ _ _ _ _ _ _ _ _ _ _ _ _ _ w486 _ _ _ _]
      tunnel: w222 -> [w235 _ _ _ _ _ w408 _ _ _ _ _ _ _ _ _ _ _ _ _ _]
      tunnel: [w234 w285 w387 w392 w401 w405 w406 w415 w425 w432 w444 w456 w463 w466 w470 w478 w485 w505 w507 w511 w524] -> w221
      tunnel: w220 -> [w234 w285 w387 w392 w401 w405 w406 _ _ w432 w444 w456 w463 w466 w470 w478 w485 w505 w507 w511 w524]
      tunnel: w219 -> [w232 _ _ _ _ _ _ _ _ _ _ _ _ _ _ _ _ _ _ _ _]
      event Timeout {
        n115 = event-data() -> ()  [unwired: 1 in, 1 out]
        n116 = local read "Mode"() -> (w237:T4)
        n117 = case shown="\"Custom\", Default" "Dashboard Tab" {
          tunnel: w240 -> [_ _ w258 _ _]
          tunnel: "TestMode/Automatic/" ("Name Pattern") -> [_ _ w257 _ _]
          tunnel: T28 [{"Operation"=enum."Clear", "Color Box"=14013909}, {"Operation"=enum."Clear", "Color Box"=14013909}, {"Operation"=enum."Clear", "Color Box"=14013909}, {"Operation"=enum."Clear", "Color Box"=14013909}, {"Operation"=enum."Update", "Color Box"=14013909}, {"Operation"=enum."Update", "Color Box"=16777215}, {"Operation"=enum."Clear", "Color Box"=14013909}, {"Operation"=enum."Clear", "Color Box"=14013909}, {"Operation"=enum."Clear", "Color Box"=14013909}] -> [_ _ w250 _ w278]
          tunnel: w237 -> [_ _ w249 _ w277]
          tunnel: u32[] [15790320, 15790320, 15790320, 15790320, 16777215, 16777215, 15790320, 15790320, 15790320] -> [_ _ _ _ w283]
          tunnel: w235 -> [_ _ _ _ w271]
          tunnel: w232 -> [_ w244 _ _ _]
          frame "Custom", Default {
            n118 = global write "Dashboard globals.vi" "Enable Vision\nProcessing"("Enable Vision\nProcessing") -> ()
            n119 = global write "Dashboard globals.vi" "Desired Target"("Desired Target") -> ()
          }
          frame "Basic" {
            n120 = call <vilib>:"WPI_DashboardUpdateNames.vi"("Controls on Tab"=w244) -> ()  [unwired: 11 in]
          }
          frame "Test" {
            w256 = -2 ("Active Item:Row Number")
            n121 = Index Array(array=w250, index=w249) -> (element=w251:T31)
            n122 = Unbundle(w251) -> ("Operation"=w252:enum16{"Update", "Clear"}, "Color Box"=w253:u32)
            n123 = call <vilib>:"NT Read String.vi"("Name"="TestMode/TestName") -> ("String"=w247:string)  [unwired: 9 in, 1 out]
            n124 = call <vilib>:"NT Read and Format Entries as Tree.vi"("Operation"=w252, "Name Pattern"=w257, "Tree Refnum"=w258) -> ()  [unwired: 7 in, 2 out]
            n125 = case shown="\"\"" w247 {
              tunnel: "TestMode/TestProgress" ("Name") -> [w260 _]
              tunnel: "TestMode/TestProgressText" ("Name") -> [w259 _]
              frame Default {
                n126 = call <vilib>:"NT Read Number.vi"("Name"=w260) -> ("Numeric"=w261:dbl)  [unwired: 9 in, 1 out]
                n127 = call <vilib>:"NT Read String.vi"("Name"=w259) -> ("String"=w262:string)  [unwired: 9 in, 1 out]
                n128 = Bundle("Numeric"=w261, "String"=w262) -> (→"Progress":cluster{"Numeric":dbl, "String":string})  [unwired: 1 in]
              }
              frame "" {
                n129 = local write "Test Name"(u16 0) -> ()
                n130 = property on="Progress" class="Clust (strict)"("Visible"=FALSE) -> ()  [unwired: 2 in, 2 out]
              }
            }
            n131 = property on="Test Tree" class="Tree (strict)"("Active Item Row Number"=w256, "ActiveColNum"=w256, "CellBG"=w253, "Active Item Row Number"=-1 ("Active Item:Row Number"), "CellBG"=u32 5789784 ("Color Box")) -> ()  [unwired: 2 in, 2 out]
          }
          frame "Variables" {
            w268 = string[] ["CameraPublisher", "Usage", "DB"]  # Items to initially close
            n132 = First Call?() -> (First Call?: T/F=w269:bool)
            n133 = control-ref of="Tree"() -> (w270:refnum<vi>)
            n134 = Select(t=w268, s=w269, f=string[] []) -> (s? t:f=w266:string[])
            n135 = call <vilib>:"NT Read and Format Entries as Tree.vi"("Tags to  Close"=w266, "Tree Refnum"=w270) -> ()  [unwired: 8 in, 2 out]
          }
          frame "Commands" {
            w279 = u32 5789784 ("Color Box")
            w280 = T32 {"Row"=-1, "Column"=-2} ("Active Cell:Active Cell")
            w282 = T32 {"Row"=-2, "Column"=-2} ("Active Cell:Active Cell")
            n136 = Index Array(array=w283, index=w277) -> (element=w281:u32)
            n137 = Index Array(array=w278, index=w277) -> (element=w276:T31)
            n138 = Unbundle(w276) -> ("Operation"=w275:enum16{"Update", "Clear"})  [unwired: 1 out]
            n139 = local read "Command Selection"() -> (w274:i32)
            n140 = property on="Command Selection" class="MCListbox (strict)"("ActiveCell"=w282, "CellBG"=w281, "ActiveCell"=w280, "CellBG"=w279) -> ()  [unwired: 2 in, 2 out]
            n141 = call <vilib>:"WPI_DashboardUpdate RPC Info.vi"("Operation"=w275) -> ("update"=w273:bool, "commands"=w272:string[][])  [unwired: 9 in]
            n142 = property on="Command Selection" class="MCListbox (strict)"("ItemNames"=w272) -> ()  [unwired: 2 in, 2 out]
            n143 = property on="Command Params" class="Tbl (strict)"("Active Cell"=w282, "Cell BG Color"=w281, "Active Cell"=w280, "Cell BG Color"=w279) -> ()  [unwired: 2 in, 2 out]
            n144 = call <vilib>:"WPI_DashboardUpdate Command Params.vi"("Update"=w273, "NewVal"=w274, "Commands"=w272, "Param Tbl"=w271) -> ()  [unwired: 7 in, 1 out]
          }
        }
        n145 = call <vilib>:"Connextion Info.vi"() -> ("Connected"=→"NT Connection":bool)  [unwired: 10 in, 1 out]
      }
      event "Test Tree": Value Change {
        # "Show appropriate\ncontrols"
        n146 = event-data() -> ("CtlRef"=w288:refnum<vi>, "NewVal"=w286:string)  [unwired: 1 in]
        n147 = call <vilib>:"WPI_UtilitiesGetTreeIOName.vi"("NewVal"=w286, "TreeControl in"=w288) -> ("I/O Name"=w289:string)  [unwired: 9 in]
        n148 = case shown="\"Camera\"" w289 {
          selector: w289 -> [_ w296 _ w318 w327 _]
          tunnel: w286 -> [_ _ w315 w317 _ w334]
          tunnel: cluster{string[]}[] [{["640x480", "320x240", "160x120"]}, {["Auto", "Fixed indoor", "Fixed outdoor 1", "Fixed outdoor 2", "Fixed fluorescent 1", "Fixed fluorescent 2", "Hold current"]}, {["Auto", "Flicker-free 50 Hz", "Flicker-free 60 Hz", "Hold current"]}, {["None", "Prioritize frame rate", "Prioritize image quality"]}, {["Monochrome", "Color"]}] -> [_ _ _ _ _ w333]
          frame Default {
            w291 = FALSE ("Visible")
            w290 = FALSE ("Visible")
            n149 = property on="Motor" class="Clust (strict)"("Visible"=w290) -> ()  [unwired: 2 in, 2 out]
            n150 = property on="Test Ring" class="Ring (strict)"("Visible"=w290) -> ()  [unwired: 2 in, 2 out]
            n151 = property on="Rev/Fwd" class="Clust (strict)"("Visible"=w291) -> ()  [unwired: 2 in, 2 out]
            n152 = property on="On/Off" class="Bool (strict)"("Visible"=w291) -> ()  [unwired: 2 in, 2 out]
            n153 = property on="Test Slider" class="Slide (strict)"("Visible"=w291) -> ()  [unwired: 2 in, 2 out]
          }
          frame "Analog Out", "Motor", "PWM" {
            w297 = FALSE ("Visible")
            n154 = case shown="\"Analog Out\"" w296 {
              tunnel: [1.0 ("Value") -1.0 ("Value") 0.0 ("Value")] -> w295
              tunnel: [255.0 ("Value") 1.0 ("Value") 5.0 ("Value")] -> w294
              tunnel: [128.0 ("Value") 0.0 ("Value") 0.0 ("Value")] -> w293
              tunnel: [64.0 ("Value") 0.5 ("Value") 1.0 ("Value")] -> w292
              frame "PWM" {
              }
              frame "Motor", Default {
              }
              frame "Analog Out" {
              }
            }
            n155 = property on="Motor" class="Clust (strict)"("Visible"=TRUE) -> ()  [unwired: 2 in, 2 out]
            n156 = property on="Value" class="Slide (strict)"("Value"=w293, "Scale.Minimum"=w295, "Scale.Maximum"=w294, "Scale.Increment"=w292) -> ()  [unwired: 2 in, 2 out]
            n157 = property on="On/Off" class="Bool (strict)"("Visible"=w297) -> ()  [unwired: 2 in, 2 out]
            n158 = property on="Test Slider" class="Slide (strict)"("Visible"=w297) -> ()  [unwired: 2 in, 2 out]
            n159 = property on="Test Ring" class="Ring (strict)"("Visible"=w297) -> ()  [unwired: 2 in, 2 out]
            n160 = property on="Rev/Fwd" class="Clust (strict)"("Visible"=w297) -> ()  [unwired: 2 in, 2 out]
          }
          frame "Servo" {
            w313 = FALSE ("Visible")
            n161 = call <vilib>:"NT Read Number.vi"("Name"=w315) -> ("Numeric"=w314:dbl)  [unwired: 9 in, 1 out]
            n162 = property on="Test Slider" class="Slide (strict)"("Visible"=TRUE, "Scale.Maximum"=170.0 ("Scale.Range:Maximum")) -> ()  [unwired: 2 in, 2 out]
            n163 = local write "Test Slider"(w314) -> ()
            n164 = property on="Motor" class="Clust (strict)"("Visible"=w313) -> ()  [unwired: 2 in, 2 out]
            n165 = property on="Rev/Fwd" class="Clust (strict)"("Visible"=w313) -> ()  [unwired: 2 in, 2 out]
            n166 = property on="On/Off" class="Bool (strict)"("Visible"=w313) -> ()  [unwired: 2 in, 2 out]
            n167 = property on="Test Ring" class="Ring (strict)"("Visible"=w313) -> ()  [unwired: 2 in, 2 out]
          }
          frame "Relay", "Solenoid" {
            w316 = FALSE ("Visible")
            n168 = property on="Motor" class="Clust (strict)"("Visible"=w316) -> ()  [unwired: 2 in, 2 out]
            n169 = property on="Test Slider" class="Slide (strict)"("Visible"=w316) -> ()  [unwired: 2 in, 2 out]
            n170 = Search and Replace String(input string=w317, search string="/Value  **", replace string="/Direction") -> (result string=w323:string)  [unwired: 5 in, 3 out]
            n171 = property on="Test Ring" class="Ring (strict)"("Visible"=w316) -> ()  [unwired: 2 in, 2 out]
            n172 = call <vilib>:"NT Read String.vi"("Name"=w323) -> ("String"=w321:string)  [unwired: 9 in, 1 out]
            n173 = Equal?(x="Both directions", y=w321) -> (x = y?=w319:bool)
            n174 = Not(x=w319) -> (.not. x?=w320:bool)
            n175 = property on="Rev/Fwd" class="Clust (strict)"("Visible"=w319) -> ()  [unwired: 2 in, 2 out]
            n176 = property on="On/Off" class="Bool (strict)"("Visible"=w320, "Caption.Text"=w318) -> ()  [unwired: 2 in, 2 out]
          }
          frame "Compressor", "Digital Out" {
            w326 = FALSE ("Visible")
            # "Get direction and finish"
            n177 = property on="Motor" class="Clust (strict)"("Visible"=w326) -> ()  [unwired: 2 in, 2 out]
            n178 = property on="Test Slider" class="Slide (strict)"("Visible"=w326) -> ()  [unwired: 2 in, 2 out]
            n179 = property on="Test Ring" class="Ring (strict)"("Visible"=w326) -> ()  [unwired: 2 in, 2 out]
            n180 = property on="On/Off" class="Bool (strict)"("Visible"=TRUE, "Caption.Text"=w327) -> ()  [unwired: 2 in, 2 out]
            n181 = property on="Rev/Fwd" class="Clust (strict)"("Visible"=FALSE) -> ()  [unwired: 2 in, 2 out]
          }
          frame "Camera" {
            n182 = call <vilib>:"Get Last Path Segment.vi"("String in"=w334) -> ("String out"=w335:string)  [unwired: 10 in]
            n183 = property on="On/Off" class="Bool (strict)"("Visible"=FALSE) -> ()  [unwired: 2 in, 2 out]
            n184 = property on="Motor" class="Clust (strict)"("Visible"=FALSE) -> ()  [unwired: 2 in, 2 out]
            n185 = property on="Rev/Fwd" class="Clust (strict)"("Visible"=FALSE) -> ()  [unwired: 2 in, 2 out]
            n186 = case shown="\"White Balance  **\"" w335 {
              tunnel: w334 -> [w341 w350 w359 w368 w377 _ w383]
              tunnel: w333 -> [w339 w347 w356 w365 w374 _ _]
              frame "Size  **" {
                n187 = Index Array(array=w339) -> (element=w338:cluster{string[]})  [unwired: 1 in]
                n188 = call <vilib>:"NT Read String.vi"("Name"=w341) -> ("String"=w340:string)  [unwired: 9 in, 1 out]
                n189 = Unbundle(w338) -> (w336:string[])
                n190 = Match First String(2:w336, 3:w340) -> (0:w337:i32)  [unwired: 1 out]
                n191 = property on="Test Ring" class="Ring (strict)"("Value"=w337, "Strings []"=w336) -> ()  [unwired: 2 in, 2 out]
                n192 = property on="Test Ring" class="Ring (strict)"("Visible"=TRUE) -> ()  [unwired: 2 in, 2 out]
                n193 = property on="Test Slider" class="Slide (strict)"("Visible"=FALSE) -> ()  [unwired: 2 in, 2 out]
              }
              frame "White Balance  **" {
                n194 = Index Array(array=w347, index=1) -> (element=w348:cluster{string[]})
                n195 = call <vilib>:"NT Read String.vi"("Name"=w350) -> ("String"=w349:string)  [unwired: 9 in, 1 out]
                n196 = Unbundle(w348) -> (w345:string[])
                n197 = Match First String(2:w345, 3:w349) -> (0:w344:i32)  [unwired: 1 out]
                n198 = property on="Test Ring" class="Ring (strict)"("Value"=w344, "Strings []"=w345) -> ()  [unwired: 2 in, 2 out]
                n199 = property on="Test Ring" class="Ring (strict)"("Visible"=TRUE) -> ()  [unwired: 2 in, 2 out]
                n200 = property on="Test Slider" class="Slide (strict)"("Visible"=FALSE) -> ()  [unwired: 2 in, 2 out]
              }
              frame "Exposure  **" {
                n201 = Index Array(array=w356, index=2) -> (element=w357:cluster{string[]})
                n202 = call <vilib>:"NT Read String.vi"("Name"=w359) -> ("String"=w358:string)  [unwired: 9 in, 1 out]
                n203 = Unbundle(w357) -> (w353:string[])
                n204 = Match First String(2:w353, 3:w358) -> (0:w354:i32)  [unwired: 1 out]
                n205 = property on="Test Ring" class="Ring (strict)"("Value"=w354, "Strings []"=w353) -> ()  [unwired: 2 in, 2 out]
                n206 = property on="Test Ring" class="Ring (strict)"("Visible"=TRUE) -> ()  [unwired: 2 in, 2 out]
                n207 = property on="Test Slider" class="Slide (strict)"("Visible"=FALSE) -> ()  [unwired: 2 in, 2 out]
              }
              frame "Exposure Priority  **" {
                n208 = Index Array(array=w365, index=3) -> (element=w366:cluster{string[]})
                n209 = call <vilib>:"NT Read String.vi"("Name"=w368) -> ("String"=w367:string)  [unwired: 9 in, 1 out]
                n210 = Unbundle(w366) -> (w362:string[])
                n211 = Match First String(2:w362, 3:w367) -> (0:w363:i32)  [unwired: 1 out]
                n212 = property on="Test Ring" class="Ring (strict)"("Value"=w363, "Strings []"=w362) -> ()  [unwired: 2 in, 2 out]
                n213 = property on="Test Ring" class="Ring (strict)"("Visible"=TRUE) -> ()  [unwired: 2 in, 2 out]
                n214 = property on="Test Slider" class="Slide (strict)"("Visible"=FALSE) -> ()  [unwired: 2 in, 2 out]
              }
              frame "Color Enable  **" {
                n215 = Index Array(array=w374, index=4) -> (element=w375:cluster{string[]})
                n216 = call <vilib>:"NT Read String.vi"("Name"=w377) -> ("String"=w376:string)  [unwired: 9 in, 1 out]
                n217 = Unbundle(w375) -> (w371:string[])
                n218 = Match First String(2:w371, 3:w376) -> (0:w372:i32)  [unwired: 1 out]
                n219 = property on="Test Ring" class="Ring (strict)"("Value"=w372, "Strings []"=w371) -> ()  [unwired: 2 in, 2 out]
                n220 = property on="Test Ring" class="Ring (strict)"("Visible"=TRUE) -> ()  [unwired: 2 in, 2 out]
                n221 = property on="Test Slider" class="Slide (strict)"("Visible"=FALSE) -> ()  [unwired: 2 in, 2 out]
              }
              frame Default {
                n222 = property on="Test Ring" class="Ring (strict)"("Visible"=FALSE) -> ()  [unwired: 2 in, 2 out]
                n223 = property on="Test Slider" class="Slide (strict)"("Visible"=FALSE) -> ()  [unwired: 2 in, 2 out]
              }
              frame "Brightness  **", "Color Level  **", "Compression  **", "FPS  **", "Sharpness  **" {
                n224 = call <vilib>:"NT Read Number.vi"("Name"=w383) -> ("Numeric"=w382:dbl)  [unwired: 9 in, 1 out]
                n225 = local write "Test Slider"(w382) -> ()
                n226 = property on="Test Slider" class="Slide (strict)"("Visible"=TRUE, "Scale.Maximum"=100.0 ("Scale.Range:Maximum")) -> ()  [unwired: 2 in, 2 out]
                n227 = property on="Test Ring" class="Ring (strict)"("Visible"=FALSE) -> ()  [unwired: 2 in, 2 out]
              }
            }
          }
        }
        n228 = property on="Progress" class="Clust (strict)"("Visible"=FALSE) -> ()  [unwired: 2 in, 2 out]
      }
      event "Test Name": Mouse Enter {
        # "Populate the ring with the list of tests"
        n229 = event-data() -> ()  [unwired: 1 in, 1 out]
        n230 = call <vilib>:"NT Read String Array.vi"("Name"="TestMode/TestList") -> ("String Array"=w391:string[])  [unwired: 9 in, 1 out]
        n231 = Build Array (concatenate)("Select the test to run...", w391) -> (w390:string[])
        n232 = property on="Test Name" class="Ring (strict)"("Strings []"=w390) -> ()  [unwired: 2 in, 2 out]
      }
      event "Test Name": Value Change {
        w393 = FALSE ("Visible")
        # "Tell the robot the test name to run"
        n233 = event-data() -> ("NewVal"=w397:u16)  [unwired: 1 in]
        n234 = property on="Test Name" class="Ring (strict)"() -> ("Strings []"=w398:string[])  [unwired: 2 in, 2 out]
        n235 = local write "Progress"(T7 {"Test Progress"=0, "Test Progress Text"=""} ("Progress")) -> ()
        n236 = Index Array(array=w398, index=w397) -> (element=w396:string)
        n237 = call <vilib>:"NT Write String.vi"("String"=w396, "Name"="TestMode/TestName") -> ()  [unwired: 9 in, 1 out]
        n238 = property on="Progress" class="Clust (strict)"("Visible"=TRUE) -> ()  [unwired: 2 in, 2 out]
        n239 = property on="Motor" class="Clust (strict)"("Visible"=w393) -> ()  [unwired: 2 in, 2 out]
        n240 = property on="Test Slider" class="Slide (strict)"("Visible"=w393) -> ()  [unwired: 2 in, 2 out]
        n241 = property on="On/Off" class="Bool (strict)"("Visible"=w393) -> ()  [unwired: 2 in, 2 out]
        n242 = property on="Rev/Fwd" class="Clust (strict)"("Visible"=w393) -> ()  [unwired: 2 in, 2 out]
        n243 = property on="Test Ring" class="Ring (strict)"("Visible"=w393) -> ()  [unwired: 2 in, 2 out]
      }
      event "Select Auto": Mouse Enter {
        # "Populate the combo box with the list of autonomous options"
        n244 = event-data() -> ()  [unwired: 1 in, 1 out]
        n245 = call <vilib>:"NT Read String Array.vi"("Name"="Auto List") -> ("String Array"=w400:string[])  [unwired: 9 in, 1 out]
        n246 = property on="Select Auto" class="CmbBox"("Strings[]"=w400) -> ()  [unwired: 2 in, 2 out]
      }
      event "Select Auto": Value Change {
        # "User modified the Auto Selection. Write to NT variable so robot knows."
        n247 = event-data() -> ("NewVal"=w403:string)  [unwired: 1 in]
        n248 = call <vilib>:"NT Write String.vi"("String"=w403, "Name"="Auto Selector") -> ()  [unwired: 9 in, 1 out]
      }
      event "Command Selection": Value Change {
        # "Get the params and show in table"
        n249 = event-data() -> ("NewVal"=w409:i32)  [unwired: 1 in]
        n250 = property on="Command Selection" class="MCListbox (strict)"() -> ("ItemNames"=w407:string[][])  [unwired: 2 in, 2 out]
        n251 = call <vilib>:"WPI_DashboardUpdate Command Params.vi"("NewVal"=w409, "Commands"=w407, "Param Tbl"=w408) -> ()  [unwired: 8 in, 1 out]
      }
      event "Execute Command": Value Change {
        # "Started one, Unique ID holds\nresponse"
        n252 = event-data() -> ()  [unwired: 1 in, 1 out]
        n253 = property on="Command Selection" class="MCListbox (strict)"() -> ("ItemNames"=w420:string[][])  [unwired: 2 in, 2 out]
        n254 = Index Array(array=w420, index (row)="Command Selection", index (col)=0) -> (element=w418:string)
        n255 = call <vilib>:"Invoke Commands.vi"("Command Params"="Command Params", "Function Name"=w418) -> ("Params"=w414:u8, "Started"=w413:bool)  [unwired: 7 in, 1 out]
        n256 = Array Subset(array="Command Params", length (row)=w414) -> (w415:string[][])  [unwired: 3 in]
        n257 = Select(t="Executing" ("Cmd Status"), s=w413, f="" ("Cmd Status")) -> (s? t:f=→"Cmd Status":string)
      }
      event "Command Selection": Double Click {
        n258 = event-data() -> ("Row"=w428:i32)  [unwired: 1 in]
        n259 = local read "Command Params"() -> (w427:string[][])
        n260 = property on="Command Selection" class="MCListbox (strict)"() -> ("ItemNames"=w431:string[][])  [unwired: 2 in, 2 out]
        n261 = Index Array(array=w431, index (row)=w428, index (col)=0) -> (element=w429:string)
        n262 = call <vilib>:"Invoke Commands.vi"("Command Params"=w427, "Function Name"=w429) -> ("Params"=w426:u8, "Started"=w421:bool)  [unwired: 7 in, 1 out]
        n263 = Array Subset(array=w427, length (row)=w426) -> (w425:string[][])  [unwired: 3 in]
        n264 = Select(t="Executing" ("Cmd Status"), s=w421, f="" ("Cmd Status")) -> (s? t:f=w422:string)
        n265 = local write "Cmd Status"(w422) -> ()
      }
      event "CheckList": Double Click {
        # "Shift clears all"
        # "Update symbols on the listbox"
        n266 = event-data() -> ("PlatMods.Shift"=w433:bool, "Row"=w435:i32)  [unwired: 1 in]
        n267 = case shown="True" w433 {
          tunnel: w435 -> [w439 _]
          tunnel: 1 -> [w438 _]
          frame False {
            n268 = property on="CheckList" class="LstBox (strict)"() -> ("Item Symbols"=w437:i32[])  [unwired: 2 in, 2 out]
            n269 = Replace Array Subset(array=w437, new element=w438, index=w439) -> (w436:i32[])
            n270 = property on="CheckList" class="LstBox (strict)"("Item Symbols"=w436) -> ()  [unwired: 2 in, 2 out]
          }
          frame True {
            w440 = 0 ("Top Row")
            n271 = property on="CheckList" class="LstBox (strict)"() -> ("Number of Rows"=w442:u32)  [unwired: 2 in, 2 out]
            n272 = Initialize Array(0, w442) -> (w441:i32[])
            n273 = property on="CheckList" class="LstBox (strict)"("Top Row"=w440, "Value"=w440, "Item Symbols"=w441) -> ()  [unwired: 2 in, 2 out]
          }
        }
      }
      event "CheckList": Key Down {
        # "Update symbols on the listbox\nLeft and right keys check and uncheck"
        n274 = event-data() -> ("VKey"=w446:T29)  [unwired: 1 in]
        n275 = case shown="\"Left\", \"Right\"" w446 {
          selector: w446 -> [w451 _]
          tunnel: eventvkey."Left" ("VKey") -> [w449 _]
          frame "Left", "Right" {
            n276 = Equal?(x=w449, y=w451) -> (x = y?=w450:bool)
            n277 = Select(t=0, s=w450, f=1) -> (s? t:f=w452:i32)
            n278 = property on="CheckList" class="LstBox (strict)"() -> ("Item Symbols"=w455:i32[])  [unwired: 2 in, 2 out]
            n279 = Replace Array Subset(array=w455, new element=w452, index="CheckList") -> (w454:i32[])
            n280 = property on="CheckList" class="LstBox (strict)"("Item Symbols"=w454) -> ()  [unwired: 2 in, 2 out]
          }
          frame Default {
          }
        }
      }
      event "Motor.Enable": Value Change {
        # "When the test mode otor enable helper is set, update that\ntree row item's value"
        n281 = event-data() -> ("NewVal"=w461:bool)  [unwired: 1 in]
        n282 = Unbundle("Motor") -> ("Value"=w460:dbl)  [unwired: 1 out]
        n283 = Select(t=w460, s=w461, f=0.0) -> (s? t:f=w458:dbl)
        n284 = call <vilib>:"NT Write Number.vi"("Numeric"=w458, "Name"=w457) -> ()  [unwired: 9 in, 1 out]
      }
      event "Test Slider": Value Change {
        # "When the test mode slider helper is set, update that\ntree row item's value"
        n285 = event-data() -> ("NewVal"=w464:dbl)  [unwired: 1 in]
        n286 = call <vilib>:"NT Write Number.vi"("Numeric"=w464, "Name"=w465) -> ()  [unwired: 9 in, 1 out]
      }
      event "On/Off": Value Change {
        # "When the test mode on/off helper value is set, update that\ntree row item's value"
        n287 = event-data() -> ("NewVal"=w469:bool)  [unwired: 1 in]
        n288 = Boolean To (0,1)(Boolean=w469) -> (0, 1=w468:i16)
        n289 = call <vilib>:"NT Write Number.vi"("Numeric"=w468, "Name"=w467) -> ()  [unwired: 9 in, 1 out]
      }
      event "Rev/Fwd": Value Change {
        # "When the test mode helper value for relays is set, update that\ntree row item's value"
        n290 = event-data() -> ("NewVal.Forward"=w477:bool, "NewVal.Reverse"=w476:bool)  [unwired: 1 in]
        n291 = Boolean To (0,1)(Boolean=w477) -> (0, 1=w473:i16)
        n292 = Boolean To (0,1)(Boolean=w476) -> (0, 1=w475:i16)
        n293 = Negate(x=w475) -> (-x=w474:i16)
        n294 = Add(x=w473, y=w474) -> (x+y=w472:i16)
        n295 = call <vilib>:"NT Write Number.vi"("Numeric"=w472, "Name"=w471) -> ()  [unwired: 9 in, 1 out]
      }
      event "Test Ring": Value Change {
        # "When a test mode helper value is selected from the ring,\nset the tree item's variable to the string value"
        n296 = event-data() -> ("NewVal"=w481:u16)  [unwired: 1 in]
        n297 = property on="Test Ring" class="Ring (strict)"() -> ("Strings []"=w482:string[])  [unwired: 2 in, 2 out]
        n298 = Index Array(array=w482, index=w481) -> (element=w480:string)
        n299 = call <vilib>:"NT Write String.vi"("String"=w480, "Name"=w479) -> ()  [unwired: 9 in, 1 out]
      }
      event "Rec Mode": Value Change {
        # "Update globals for recording mode and path to read log from.\nClear when logging and let NetworkTables set path for vision to\nuse."
        n300 = event-data() -> ("NewVal"=w493:enum32{"Stop", "Record", "Playback"})  [unwired: 1 in]
        n301 = global write "WPI_DashboardLogging Global.vi" "Logging Filename"(path "") -> ()
        n302 = global write "WPI_DashboardLogging Global.vi" "Recording"(w493) -> ()
        n303 = case shown="\"Playback\"" w493 {
          tunnel: w492 -> [_ w495 w504]
          tunnel: [_ _ w503] -> w490
          tunnel: [_ _ w502] -> _
          tunnel: w488 -> [_ _ w500]
          tunnel: cluster{i32, i32} {-250, 170} -> [_ _ w499]
          tunnel: [_ _ T30 {"Image Size"=TRUE, "Image Type"=TRUE, "Pixel Value"=TRUE, "ROI Information"=TRUE, "Zoom Factor"=FALSE} ("Image Information Shown:All Elements")] -> w483
          tunnel: [_ _ TRUE ("Zoom Factor")] -> w484
          tunnel: w486 -> [_ _ w496]
          frame Default {
          }
          frame "Stop", "Record" {
            # "Place Window too"
            n304 = invoke class="VI" method="FP.Close"(reference=w495) -> (reference out=w494:refnum<vi>)  [unwired: 2 in, 2 out]
            n305 = invoke class="VI" method="Abort VI"(reference=w494) -> ()  [unwired: 2 in, 3 out]
          }
          frame "Playback" {
            n306 = call "Open Playback Panel.vi"("Offset"=w499, "DB VI Ref"=w500, "Playback in"=w504) -> ("Playback out"=w501:refnum<vi>)  [unwired: 8 in]
            n307 = register-events(w501, w496) -> (reference out=w503:refnum<event-registration>, error out=w502:errorcluster)  [unwired: 2 in]
          }
        }
        n308 = property on="Camera Image Right" class="ImageControl"("Image Information Shown"=w483, "Image Information Visible"=w484) -> ()  [unwired: 2 in, 2 out]
        n309 = property on="Camera Image" class="ImageControl"("Image Information Shown"=w483, "Image Information Visible"=w484) -> ()  [unwired: 2 in, 2 out]
        n310 = call <vilib>:"WPI_DashboardNT Log FieldName Cache.vi"("Operation"=enum16{"Lookup/Add", "Index", "Clear"}."Clear") -> ()  [unwired: 8 in, 3 out]
      }
      event Panel Close {
        w506 = enum32{"Stop", "Record", "Playback"}."Stop" ("Rec Mode")
        # "Playback window has been closed, abort"
        n311 = event-data() -> ()  [unwired: 1 in, 4 out]
        n312 = local write "Rec Mode"(w506) -> ()
        n313 = global write "WPI_DashboardLogging Global.vi" "Recording"(w506) -> ()
      }
      event Panel Close {
        # "Abort playback window and ourself"
        n314 = event-data() -> ()  [unwired: 1 in, 4 out]
        n315 = invoke class="VI" method="FP.Close"(reference=w510) -> (reference out=w509:refnum<vi>)  [unwired: 2 in, 2 out]
        n316 = invoke class="VI" method="Abort VI"(reference=w509) -> (error out=w508:errorcluster)  [unwired: 2 in, 2 out]
        n317 = invoke class="VI" method="Abort VI"(error in=w508) -> ()  [unwired: 2 in, 3 out]
      }
      event User Event {
        n318 = event-data() -> ("IDs"=w517:cluster{"RPC field ID":u16, "Unique ID":u16}, "String"=w516:string)  [unwired: 1 in]
        n319 = Bundle("IDs"=w517, "String"=w516) -> (w515:T10)  [unwired: 1 in]
        n320 = call <vilib>:"Retrieve RPC Response.vi"("RPC Response"=w515) -> ("Output"=w513:string[][])  [unwired: 10 in]
        n321 = Build Array (concatenate)(w511, w513) -> (w512:string[][])
        n322 = local write "Command Params"(w512) -> ()
        n323 = local write "Cmd Status"("" ("Cmd Status")) -> ()
      }
      event "Tree": Double Click {
        n324 = event-data() -> ("PlatMods"=w523:T33, "Tag"=w520:string)  [unwired: 1 in]
        n325 = Unbundle(w523) -> ("Shift"=w522:bool)  [unwired: 4 out]
        n326 = String Subset(string=w520, length (rest)=1 ("length (rest)")) -> (substring=w519:string)  [unwired: 1 in]
        n327 = Not(x=w522) -> (.not. x?=w521:bool)
        n328 = case shown="\"/\"" w519 {
          tunnel: w520 -> [_ w526]
          tunnel: w521 -> [_ w525]
          frame Default {
          }
          frame "/" {
            n329 = call <vilib>:"NT Update Persistence.vi"("Persistence"=w525, "Name"=w526) -> ()  [unwired: 9 in, 1 out]
          }
        }
      }
    }
  }
  n330 = while {
    tunnel: w66 -> [w528]
    i -> [w531]
    stop <- FALSE stop-if-true
    n331 = Wait (ms)(milliseconds to wait=u32 100) -> ()  [unwired: 1 out]
    n332 = case shown="\"Playback\"" "Rec Mode" {
      tunnel: w531 -> [_ _ w546]
      tunnel: [u32 2829099 ("Base Color") u32 11141120 ("Target Color") w535] -> w527
      frame "Stop", Default {
        # "Reset the color, extra updates don't cost much"
      }
      frame "Record" {
      }
      frame "Playback" {
        # "Playback"
        n333 = Quotient & Remainder(x=w546, y=u32 50 ("milliseconds to wait")) -> (x-y*floor(x/y)=w542:u32)  [unwired: 1 out]
        n334 = Divide(x=w542, y=u32 50 ("milliseconds to wait")) -> (x/y=w539:dbl)
        n335 = Multiply(x=6.283185307179586, y=w539) -> (x*y=w544:dbl)
        n336 = Sine(x=w544) -> (sin(x)=w543:dbl)
        n337 = Absolute Value(x=w543) -> (abs(x)=w536:dbl)
        n338 = call "Interpolate RGB Color.vi"("Proportion"=w536, "Target Color"=u32 30976, "Base Color"=u32 2829099) -> ("Result Color"=w535:u32)  [unwired: 8 in]
      }
    }
    n339 = property class="Pane"(reference=w528, "PaneColor"=w527) -> ()  [unwired: 1 in, 2 out]
  }
  n340 = local write "Dashboard Tab"(T2."Drive" ("Dashboard Tab")) -> ()
  n341 = property on="On/Off" class="Bool (strict)"("Visible"=w37) -> ()  [unwired: 2 in, 2 out]
  n342 = property on="Motor" class="Clust (strict)"("Visible"=w37) -> ()  [unwired: 2 in, 2 out]
  n343 = property on="Progress" class="Clust (strict)"("Visible"=w37) -> ()  [unwired: 2 in, 2 out]
  n344 = property on="Test Ring" class="Ring (strict)"("Visible"=w37) -> ()  [unwired: 2 in, 2 out]
  n345 = property on="Rev/Fwd" class="Clust (strict)"("Visible"=w37) -> ()  [unwired: 2 in, 2 out]
  n346 = while {
    tunnel: u16 1741 ("timeout ms (25000)") -> [w548]
    stop <- FALSE stop-if-true
    n347 = TCP Create Listener(10:w548) -> (0:w547:errorcluster, 3:w549:refnum<k5>)  [unwired: 4 in, 1 out]
    n348 = case shown="No Error" w547 {
      selector: w547 -> [w551 _]
      tunnel: w549 -> [w552 _]
      frame No Error {
        n349 = while {
          tunnel: w552 -> [w555]
          tunnel: w551 -> [w554]
          stop <- FALSE stop-if-true
          n350 = TCP Wait On Listener(8:w554, 11:w555) -> (0:w556:errorcluster, 4:w557:refnum<k5>)  [unwired: 2 in, 3 out]
          n351 = local write "TCP"(w557) -> ()
          n352 = case shown="No Error" w556 {
            frame No Error {
            }
            frame Error {
              n353 = Wait (ms)(milliseconds to wait=u32 1000) -> ()  [unwired: 1 out]
            }
          }
        }
      }
      frame Error {
        n354 = Wait (ms)(milliseconds to wait=u32 1000) -> ()  [unwired: 1 out]
      }
    }
  }
  n355 = local write "Command Selection"(u16 0 ("milliseconds to wait")) -> ()
  n356 = local write "Command Params"(string[][] [] ("Command Params")) -> ()
  n357 = global write "WPI_DashboardLogging Global.vi" "Recording"(w60) -> ()
  n358 = local write "Rec Mode"(w60) -> ()
  n359 = call <vilib>:"NT Write String.vi"("String"="Select Auto", "Name"="Auto Selector") -> ()  [unwired: 9 in, 1 out]
